vi "Combine Channel Output.vi"(8 "error in (no error)":errorcluster, 9 "Source Channel (0: None)":i32(ring) items=["1"=1, "2"=2, "None"=0], 10 "Base Channel (1:1)":i32(ring)=1 items=["1"=1, "2"=2], 11 "VISA resource name":refnum<visa-resource-name>) -> (0 "error out":errorcluster, 3 "VISA resource name out":refnum<visa-resource-name>)   [LabVIEW 2013, in "AWG.lvlib" / "Agilent 3352X Series.lvlib"]
doc: "Allows digital data from both channels to added together to create the output signal on the output DAC for the base channel. \nCan be used to (1) generate quadrature modulated signals from the two channels to be added together into a single connector (2) add noise from a second channel to a modulated signal on the base channel. \n\n<b>Note</b>:\n(1) Only one channel may operate in combine mode at a time \n(2) Set up both channels for their respective signal frequency, amplitude, modulation, and so forth before combine them together. \n(3) Signals are combined in digital form.The lower amplitude signal may have reduced resolution proportional to the ratio of the two amplitudes. \n(4) When signals are combined, their peak amplitude may not exceed the output rating for the waveform generator or the programmed limits."
uses:
  Agilent 3352X Series.lvlib
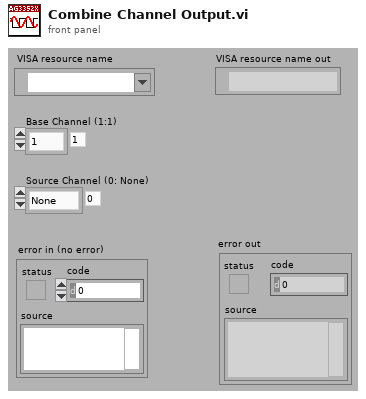
[diagram p1: front panel]
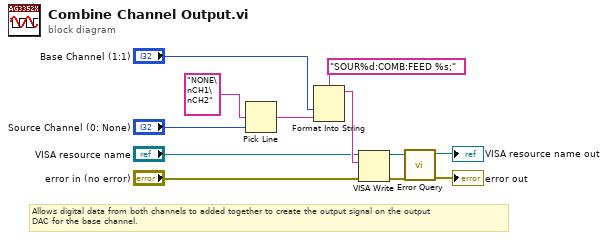
[diagram p0: block diagram]
diagram:
  # "Allows digital data from both channels to added together to create the output signal on the output \nDAC for the base channel."
  n1 = Pick Line(multi-line string="NONE\nCH1\nCH2", line index="Source Channel (0: None)") -> (output string=w6:string)  [unwired: 1 out]
  n2 = Format Into String(format string="SOUR%d:COMB:FEED %s;", "Base Channel (1:1)", w6) -> (resulting string=w10:string)  [unwired: 2 in, 1 out]
  n3 = VISA Write(VISA resource name="VISA resource name", write buffer=w10, error in (no error)="error in (no error)") -> (VISA resource name out=w4:refnum<visa-resource-name>, error out=w2:errorcluster)  [unwired: 1 out]
  n4 = call "Error Query.vi"("error in (no error)"=w2, "VISA resource name"=w4) -> ("error out"=→"error out":errorcluster, "VISA resource name out"=→"VISA resource name out":refnum<visa-resource-name>)  [unwired: 8 out]
